vi "Sample Transfer Set Timeout.vi"(8 "error in (no error)":errorcluster, 10 "Sample Transfer.State Timeout (0)":dbl, 11 "cRIO-CO2 in":refnum<class "cRIO-CO2.lvclass">) -> (0 "error out":errorcluster, 3 "cRIO-CO2 out":refnum<class "cRIO-CO2.lvclass">)   [LabVIEW 2015, in "cRIO-Carbondioxide.lvlib" / "cRIO-CO2.lvlib" / "cRIO-CO2.lvclass"]
uses:
  cRIO-CO2.lvclass
  cRIO-CO2.lvclass/cRIO-CO2.ctl
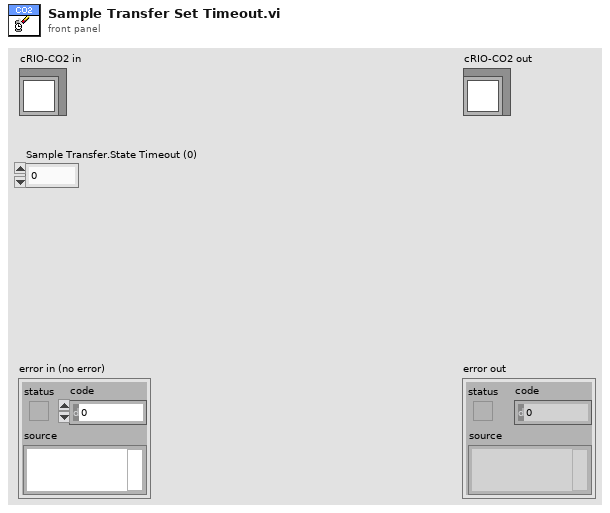
[diagram p1: front panel]
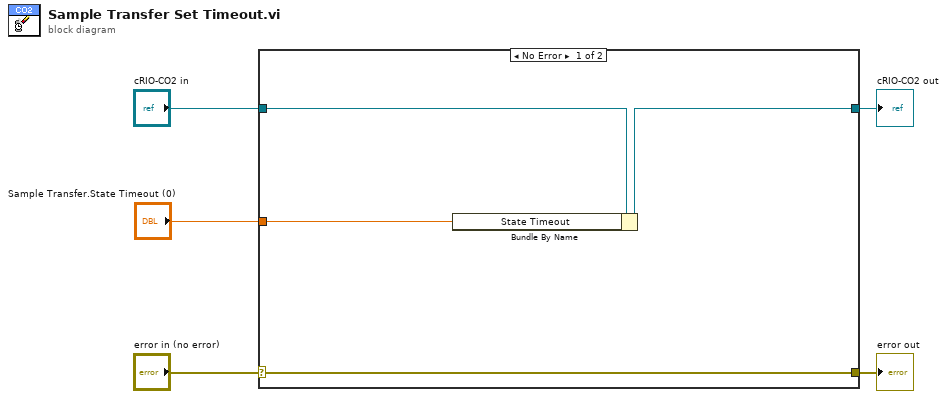
[diagram p0: block diagram]
diagram:
  n1 = case shown="No Error" "error in (no error)" {
    selector: "error in (no error)" -> [w8 w11]
    tunnel: [w8 w11] -> w4
    tunnel: [w7 w10] -> w2
    tunnel: "cRIO-CO2 in" -> [w9 w10]
    tunnel: "Sample Transfer.State Timeout (0)" -> [w6 _]
    frame No Error {
      n2 = Bundle By Name(cluster=w9, "State Timeout"=w6) -> (w7:refnum<class "cRIO-CO2.lvclass">)
    }
    frame Error {
    }
  }
  "error out" <- w4
  "cRIO-CO2 out" <- w2
